vi "CCD3000 Spectral Acquisition.vi"(5 "Acquire":refnum<vi>, 7 "Running":refnum<vi>, 11 "Comm Params":T1={"Comm Interface"=1, "BUS"=0, "Address"=5, "Com Port"=1} {"Comm Interface" items=["RS 232", "GPIB"]}) -> (0 "error out":errorcluster, 2 "Raw-Spectrum":u16[](array[numeric]), 3 "Data":u16[][](array[numeric]))   [LabVIEW 2010]
uses:
  drivers/Horiba Spectrum One 3000V/Lib/CCD_command.llb/Comm Params.ctl
panel:
  out "Data":u32
  out "Stop":u32
  out "Readout":u32
  out "Polling":u32
  out "Initiate":u32
  in  "CCD ADC and Gain":dbl(ring) items=["16 bits Gain 1", "16 bits Gain 2", "16 bits Gain 3", "16 bits Gain 4", "14 bits Gain 1", "14 bits Gain 2"]
  out "Waveform Graph":u16[](graph)
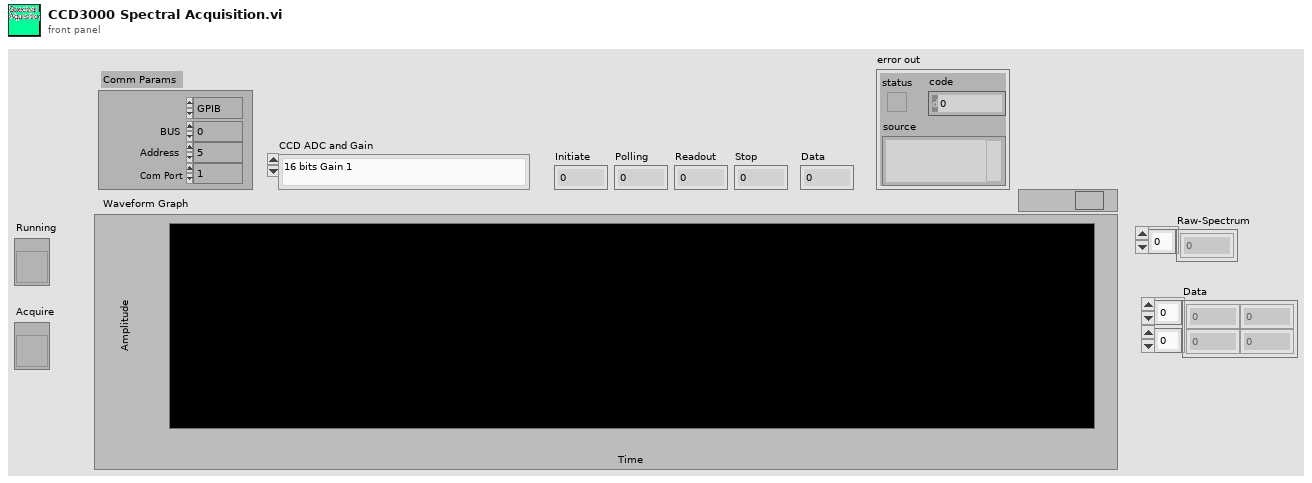
[diagram p1: front panel]
types:
  T1 = typedef "Comm Params.ctl" = cluster{"Comm Interface":u16, "BUS":i16, "Address":i16, "Com Port":i32}
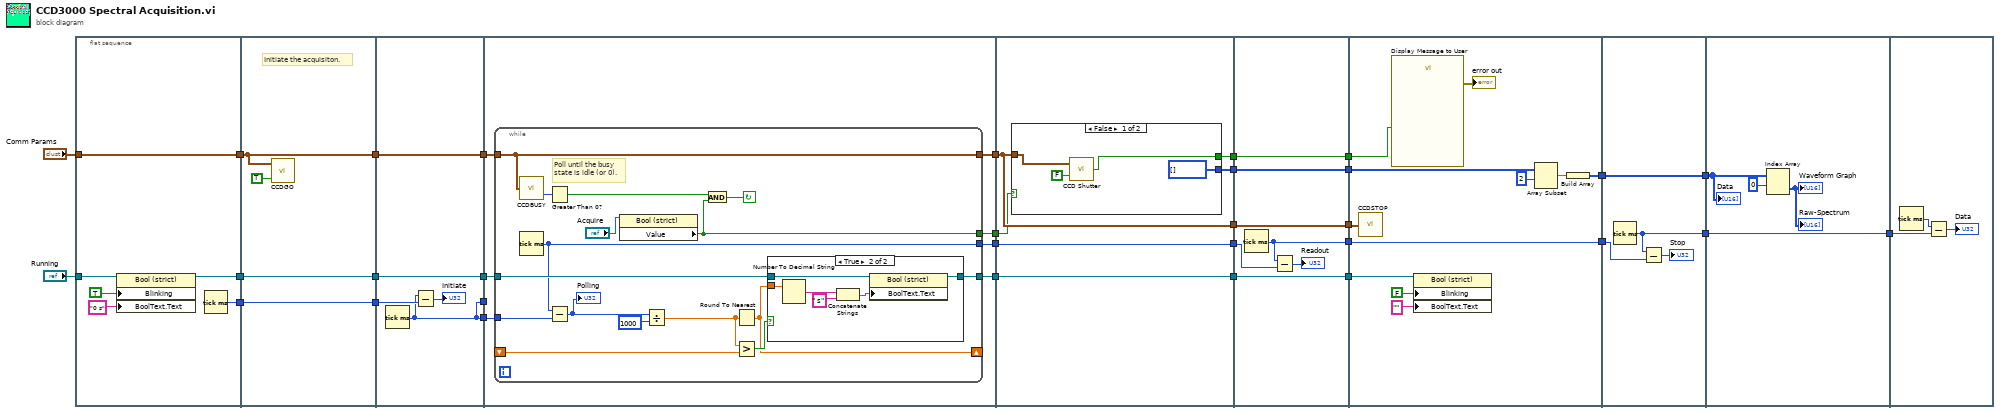
[diagram p0: block diagram]
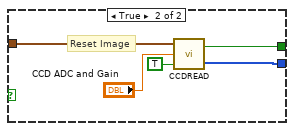
[diagram p3: hidden frame]
diagram:
  n1 = flat-sequence {
    tunnel: "Comm Params" -> [w37]
    tunnel: [w37] -> w30
    tunnel: "Running" -> [w36]
    tunnel: [w34] -> w28
    tunnel: [w33] -> w27
    tunnel: [w40] -> w18
    tunnel: w30 -> [w40]
    tunnel: w28 -> [w39]
    tunnel: [w39] -> w16
    tunnel: w27 -> [w38]
    tunnel: [w38] -> w14
    tunnel: w18 -> [w46]
    tunnel: [w46] -> w17
    tunnel: w16 -> [w45]
    tunnel: [w45] -> w15
    tunnel: w14 -> [w43]
    tunnel: [w42] -> w6
    tunnel: [w42] -> w5
    tunnel: w17 -> [w53]
    tunnel: [w52] -> w4
    tunnel: w15 -> [w50]
    tunnel: [w49] -> w3
    tunnel: [w51] -> w2
    tunnel: w6 -> [_]
    tunnel: w5 -> [w48]
    tunnel: [w47] -> w1
    tunnel: w4 -> [w81]
    tunnel: [w82] -> w26
    tunnel: [w81] -> w24
    tunnel: w3 -> [w80]
    tunnel: [w80] -> w22
    tunnel: w2 -> [w79]
    tunnel: [w78] -> w20
    tunnel: w1 -> [w77]
    tunnel: [w77] -> w7
    tunnel: w26 -> [w98]
    tunnel: [w98] -> w25
    tunnel: w24 -> [w97]
    tunnel: [w97] -> w23
    tunnel: w22 -> [w96]
    tunnel: [w96] -> w21
    tunnel: w20 -> [w95]
    tunnel: [w95] -> w19
    tunnel: [w93] -> w9
    tunnel: w7 -> [w92]
    tunnel: w25 -> [w104]
    tunnel: w23 -> [w109]
    tunnel: w21 -> [w105]
    tunnel: w19 -> [w107]
    tunnel: [w101] -> w13
    tunnel: w9 -> [w100]
    tunnel: [w100] -> w8
    tunnel: w13 -> [w113]
    tunnel: [w113] -> w12
    tunnel: [w111] -> w11
    tunnel: w8 -> [w110]
    tunnel: w12 -> [w115]
    tunnel: w11 -> [w117]
    tunnel: [w117] -> w10
    tunnel: w10 -> [w118]
    frame #0 {
      n2 = property class="Bool (strict)"(reference=w36, "Blinking"=TRUE ("Blinkend"), "BoolText.Text"="0 s" ("Boolean Text.Text")) -> (reference out=w34:refnum<vi>)  [unwired: 1 in, 1 out]
      n3 = Tick Count (ms)() -> (millisecond timer value=w33:u32)
    }
    frame #1 {
      # "Initiate the acquisiton."
      n4 = call "CCDGO.VI"("Shutter"=TRUE ("Use Shutter"), "Comm Params"=w40) -> ()  [unwired: 1 in, 1 out]
    }
    frame #2 {
      n5 = Tick Count (ms)() -> (millisecond timer value=w42:u32)
      n6 = Subtract(x=w42, y=w43) -> (x-y=→"Initiate":u32)
    }
    frame #3 {
      n7 = while {
        tunnel: w53 -> [w68]
        tunnel: [w68] -> w52
        tunnel: [w64] -> w51
        tunnel: w50 -> [w63]
        tunnel: [w62] -> w49
        shift-right: [w57] -> _
        shift-left: _ -> [w59]
        tunnel: w48 -> [w56]
        tunnel: [w55] -> w47
        stop <- w67 continue-if-true
        # "Poll until the busy\nstate is idle (or 0)."
        n8 = call "CCDBUSY.VI"("Comm Params"=w68) -> ("CCD Status"=w69:u16)  [unwired: 1 out]
        n9 = Tick Count (ms)() -> (millisecond timer value=w55:u32)
        n10 = Greater Than 0?(x=w69) -> (x > 0?=w66:bool)
        n11 = Subtract(x=w55, y=w56) -> (x-y=w54:u32)
        "Polling" <- w54
        n12 = property class="Bool (strict)"(reference="Acquire") -> ("Value"=w64:bool)  [unwired: 1 in, 2 out]
        n13 = Divide(x=w54, y=u32 1000) -> (x/y=w58:dbl)
        n14 = And(x=w66, y=w64) -> (x .and. y?=w67:bool)
        n15 = Round To Nearest(number=w58) -> (nearest integer value=w57:dbl)
        n16 = Greater?(x=w58, y=w59) -> (0:w60:bool)
        n17 = case shown="True" w60 {
          tunnel: w63 -> [w70 w76]
          tunnel: [w70 w75] -> w62
          tunnel: w57 -> [_ w71]
          frame False {
          }
          frame True {
            n18 = Number To Decimal String(number=w71) -> (decimal integer string=w74:string)  [unwired: 1 in]
            n19 = Concatenate Strings(w74, " s" ("string")) -> (w73:string)
            n20 = property class="Bool (strict)"(reference=w76, "BoolText.Text"=w73) -> (reference out=w75:refnum<vi>)  [unwired: 1 in, 1 out]
          }
        }
      }
    }
    frame #4 {
      n21 = case shown="False" w79 {
        tunnel: [w83 w90] -> w78
        tunnel: [u16[] [] ("Data") w89] -> w82
        tunnel: w81 -> [w85 w87]
        frame False {
          n22 = call "CCD Shutter.vi"("Shutter"=FALSE, "Comm Params"=w85) -> ("Error"=w83:bool)
        }
        frame True {
          # "Reset Image"
          n23 = call "CCDREAD.VI"("Reset Image?"=TRUE, "CCD ADC and Gain"="CCD ADC and Gain", "Comm Params"=w87) -> ("Data"=w89:u16[], "Error"=w90:bool)
        }
      }
    }
    frame #5 {
      n24 = Tick Count (ms)() -> (millisecond timer value=w93:u32)
      n25 = Subtract(x=w93, y=w92) -> (x-y=→"Readout":u32)
    }
    frame #6 {
      n26 = call "CCDSTOP.VI"("Comm Params"=w109) -> ()  [unwired: 1 out]
      n27 = call "Display Message to User"("Enable"=w107) -> ("error out"=→"error out":errorcluster)  [unwired: 9 in, 1 out]
      n28 = property class="Bool (strict)"(reference=w105, "Blinking"=FALSE ("Blinkend"), "BoolText.Text"="" ("Boolean Text.Text")) -> ()  [unwired: 1 in, 2 out]
      n29 = Array Subset(array=w104, index=2) -> (w102:u16[])  [unwired: 1 in]
      n30 = Build Array(w102) -> (w101:u16[][])
    }
    frame #7 {
      n31 = Tick Count (ms)() -> (millisecond timer value=w111:u32)
      n32 = Subtract(x=w111, y=w110) -> (x-y=→"Stop":u32)
    }
    frame #8 {
      n33 = Index Array(array=w115, index (row)=0 ("Index (Zeile)")) -> (element=→"Waveform Graph" →"Raw-Spectrum":u16[])  [unwired: 1 in]
      "Data" <- w115
    }
    frame #9 {
      n34 = Tick Count (ms)() -> (millisecond timer value=w119:u32)
      n35 = Subtract(x=w119, y=w118) -> (x-y=→"Data":u32)
    }
  }
